vi "Disconnect.vi"(8 "error in (no error)":errorcluster, 11 "OXY_SCPI Reseource Out":refnum<visa-resource-name>) -> (0 "error out":errorcluster)   [LabVIEW 2018, in "OXYGEN.lvlib"]
uses:
  OXYGEN.lvlib
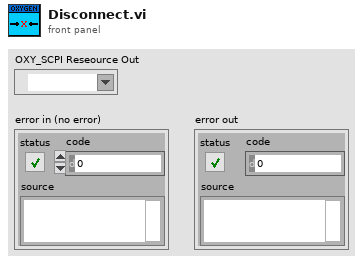
[diagram p1: front panel]
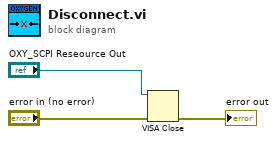
[diagram p0: block diagram]
diagram:
  n1 = VISA Close(VISA resource name="OXY_SCPI Reseource Out", error in (no error)="error in (no error)") -> (error out=→"error out":errorcluster)
